vi "SensorDAQ.vi"(8 "error in (no error)":errorcluster, 9 "Message Notifiers":T1, 10 "UI Queue":refnum<queue>, 11 "Logging Queue":refnum<queue>) -> (0 "error out":errorcluster)   [LabVIEW 2018]
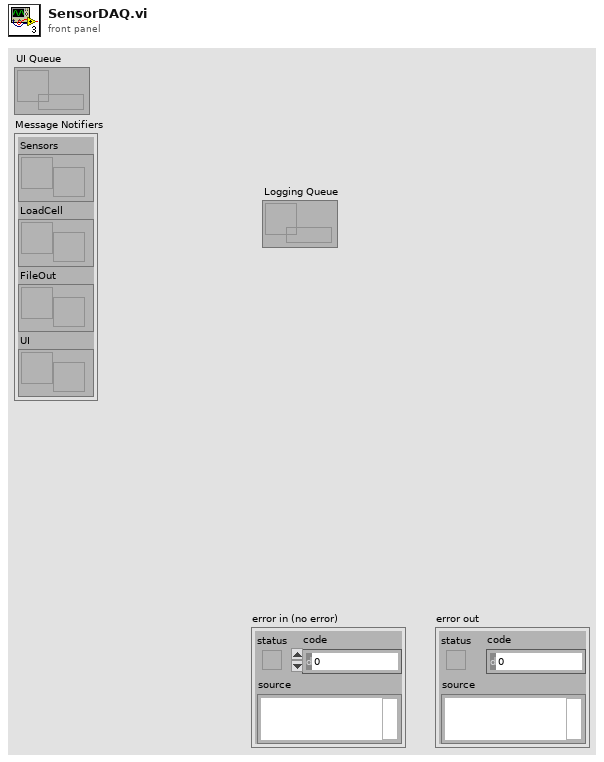
[diagram p1: front panel]
types:
  T1 = cluster{"Sensors":refnum<notifier>, "LoadCell":refnum<notifier>, "FileOut":refnum<notifier>, "UI":refnum<notifier>}
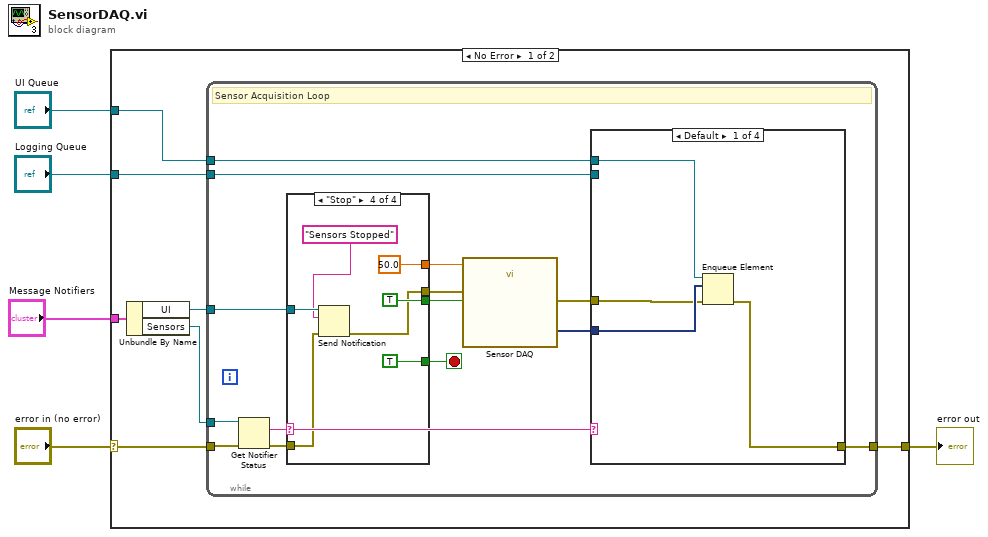
[diagram p0: block diagram]
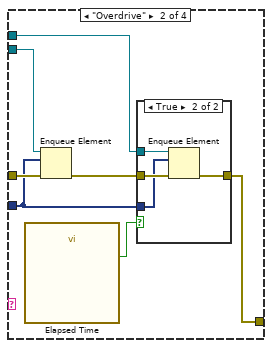
[diagram p2: hidden frame]
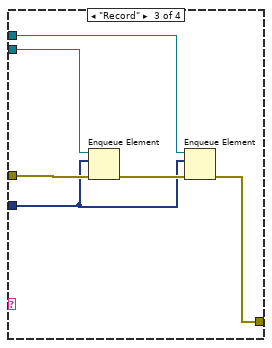
[diagram p4: hidden frame]
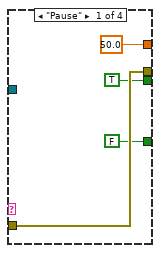
[diagram p6: hidden frame]
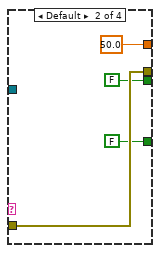
[diagram p7: hidden frame]
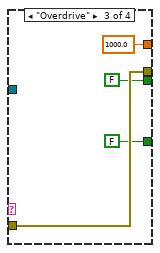
[diagram p8: hidden frame]
diagram:
  n1 = case shown="No Error" "error in (no error)" {
    selector: "error in (no error)" -> [w10 w69]
    tunnel: "Message Notifiers" -> [w12 _]
    tunnel: [w6 w69] -> w4
    tunnel: "Logging Queue" -> [w8 _]
    tunnel: "UI Queue" -> [w7 _]
    frame No Error {
      n2 = Unbundle By Name(w12) -> ("UI"=w11:refnum<notifier>, "Sensors"=w9:refnum<notifier>)
      n3 = while {
        tunnel: w11 -> [w22]
        tunnel: w10 -> [w13]
        tunnel: w9 -> [w14]
        tunnel: w8 -> [w18]
        tunnel: w7 -> [w17]
        tunnel: [w20] -> w6
        stop <- w23 stop-if-true
        # "Sensor Acquisition Loop"
        n4 = Get Notifier Status(notifier=w14, error in (no error)=w13) -> (current notification=w16:string, error out=w15:errorcluster)  [unwired: 3 out]
        n5 = case shown="\"Stop\"" w16 {
          tunnel: [TRUE FALSE FALSE TRUE] -> w26
          tunnel: [w52 w56 w60 w64] -> w25
          tunnel: [50.0 50.0 1000.0 50.0] -> w24
          tunnel: w15 -> [w52 w56 w60 w62]
          tunnel: [FALSE FALSE FALSE TRUE] -> w23
          tunnel: w22 -> [_ _ _ w65]
          frame "Pause" {
          }
          frame Default {
          }
          frame "Overdrive" {
          }
          frame "Stop" {
            n6 = Send Notification(notification="Sensors Stopped", notifier=w65, error in (no error)=w62) -> (error out=w64:errorcluster)  [unwired: 1 out]
          }
        }
        n7 = call "Sensor DAQ"("rate"=w24, "error in"=w25, "stop (F)"=w26) -> ("data"=w21:dynamicdata, "error out"=w19:errorcluster)  [unwired: 13 in, 2 out]
        n8 = case shown="Default" w16 {
          tunnel: w21 -> [w29 w32 w44 _]
          tunnel: [w27 w33 w43 w49] -> w20
          tunnel: w19 -> [w28 w37 w48 w49]
          tunnel: w18 -> [_ w36 w47 _]
          tunnel: w17 -> [w30 w35 w46 _]
          frame Default {
            n9 = Enqueue Element(queue=w30, element=w29, error in (no error)=w28) -> (error out=w27:errorcluster)  [unwired: 1 in, 2 out]
          }
          frame "Overdrive" {
            n10 = call "Elapsed Time"() -> ("Time has Elapsed"=w31:bool)  [unwired: 12 in, 7 out]
            n11 = Enqueue Element(queue=w36, element=w32, error in (no error)=w37) -> (error out=w34:errorcluster)  [unwired: 1 in, 2 out]
            n12 = case shown="True" w31 {
              tunnel: w35 -> [_ w42]
              tunnel: w34 -> [w38 w41]
              tunnel: [w38 w40] -> w33
              tunnel: w32 -> [_ w39]
              frame False {
              }
              frame True {
                n13 = Enqueue Element(queue=w42, element=w39, error in (no error)=w41) -> (error out=w40:errorcluster)  [unwired: 1 in, 2 out]
              }
            }
          }
          frame "Record" {
            n14 = Enqueue Element(queue=w47, element=w44, error in (no error)=w48) -> (error out=w45:errorcluster)  [unwired: 1 in, 2 out]
            n15 = Enqueue Element(queue=w46, element=w44, error in (no error)=w45) -> (error out=w43:errorcluster)  [unwired: 1 in, 2 out]
          }
          frame "Pause", "Stop" {
          }
        }
      }
    }
    frame Error {
    }
  }
  "error out" <- w4
